vi "rtp play.vi"(4 "voltage range":dbl, 6 "freq":u32, 7 "rtp stop event ref":refnum<user-event>, 8 "error in (no error)":errorcluster caption="에러 입력(에러 없음)", 10 "waveform data":i8[](array[numeric]), 11 "DW7914 입력":refnum<class "DW7914.lvclass">) -> (0 "error out":errorcluster caption="에러 출력", 3 "DW7914 출력":refnum<class "DW7914.lvclass">)   [LabVIEW 2020, in "DW7914.lvclass"]
uses:
  DW7914.lvclass
  Haptic IC/Haptic IC.lvclass/Haptic IC.ctl
  SubVIs/I2C/Instance VIs/(SubVI)I2C_8Bit-8Bit_Read_Single.vi
  SubVIs/I2C/Instance VIs/(SubVI)I2C_8Bit-8Bit_Write_Single.vi
  DW7912/DW7912.lvclass
  Haptic IC/Haptic IC.lvclass
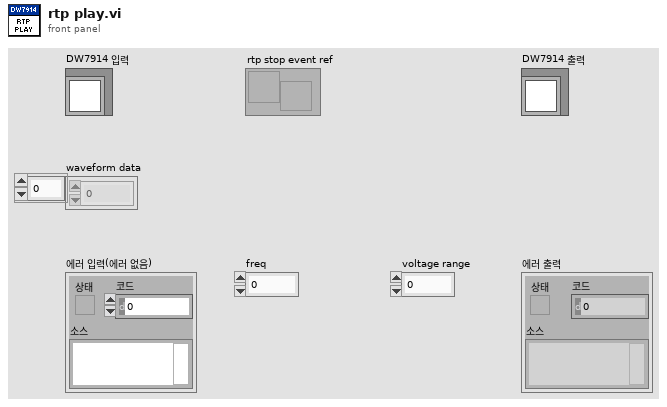
[diagram p1: front panel]
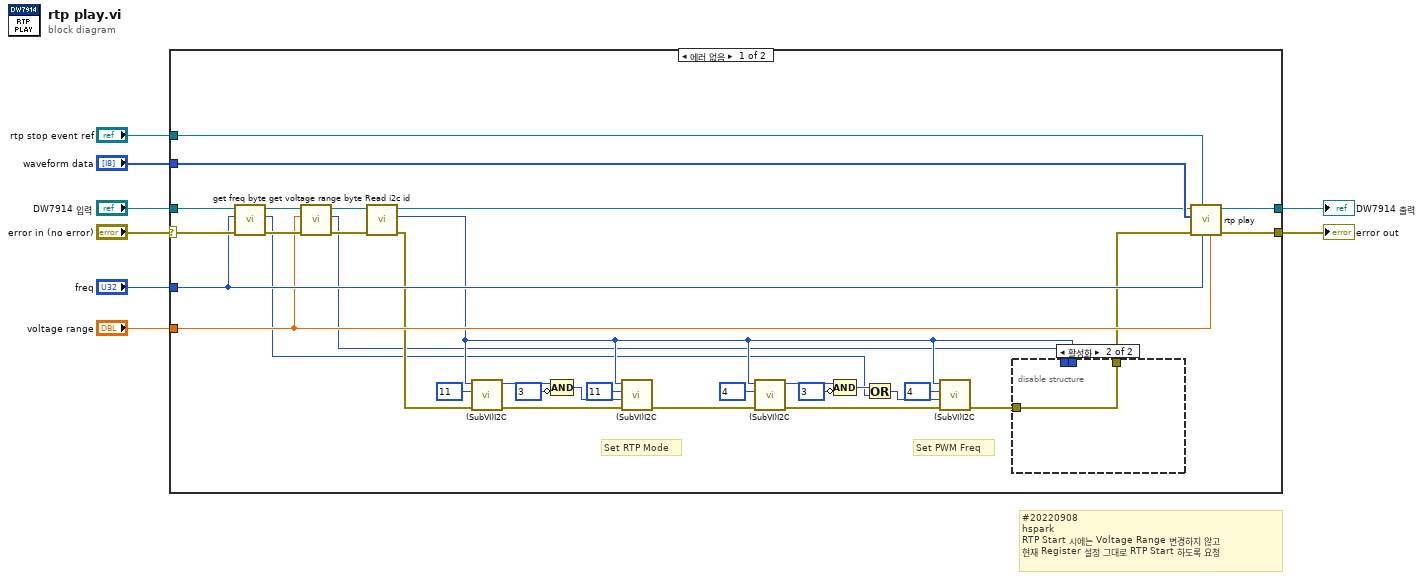
[diagram p0: block diagram]
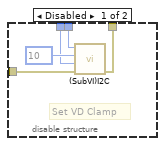
[diagram p2: hidden frame]
diagram:
  # "#20220908\nhspark\nRTP Start 시에는 Voltage Range 변경하지 않고\n현재 Register 설정 그대로 RTP Start 하도록 요청"
  n1 = case shown="에러 없음" "error in (no error)" {
    selector: "error in (no error)" -> [w38 w48]
    tunnel: [w41 w48] -> w8
    tunnel: [w40 w49] -> w7
    tunnel: "voltage range" -> [w32 _]
    tunnel: "freq" -> [w33 _]
    tunnel: "rtp stop event ref" -> [w39 _]
    tunnel: "DW7914 입력" -> [w36 w49]
    tunnel: "waveform data" -> [w37 _]
    frame No Error {
      # "Set PWM Freq"
      # "Set RTP Mode"
      n2 = call-dynamic "get freq byte.vi"("error in (no error)"=w38, "freq"=w33, "DW7912 입력"=w36) -> ("error out"=w35:errorcluster, "byte value"=w10:u8, "DW7912 출력"=w34:refnum<class "DW7914.lvclass">)  [unwired: 6 in]
      n3 = call-dynamic "get voltage range byte.vi"("error in (no error)"=w35, "voltage range"=w32, "DW7912 입력"=w34) -> ("error out"=w31:errorcluster, "byte value"=w9:u8, "DW7912 출력"=w30:refnum<class "DW7914.lvclass">)  [unwired: 6 in]
      n4 = call "Read i2c id.vi"("error in (no error)"=w31, "Haptic IC 입력"=w30) -> ("error out"=w28:errorcluster, "i2c id"=w13:u8, "Haptic IC 출력"=w29:refnum<class "DW7914.lvclass">)  [unwired: 7 in]
      n5 = call-poly "(SubVI)I2C.vi"("error in (no error)"=w28, "Address"=u8 11, "ID"=w13) -> ("error out"=w23:errorcluster, "Read Data"=w26:u8)  [unwired: 6 in, 1 out]
      n6 = Compound Arithmetic op=AND(w26, invert u8 3 ("y")) -> (w22:u8)
      n7 = call-poly "(SubVI)I2C.vi"("error in (no error)"=w23, "Data to Write"=w22, "Address"=u8 11, "ID"=w13) -> ("error out"=w16:errorcluster)  [unwired: 6 in, 1 out]
      n8 = call-poly "(SubVI)I2C.vi"("error in (no error)"=w16, "Address"=u8 4, "ID"=w13) -> ("error out"=w20:errorcluster, "Read Data"=w18:u8)  [unwired: 6 in, 1 out]
      n9 = Compound Arithmetic op=AND(w18, invert u8 3 ("y")) -> (w21:u8)
      n10 = Or(x=w21, y=w10) -> (x .or. y?=w11:u8)
      n11 = call-poly "(SubVI)I2C.vi"("error in (no error)"=w20, "Data to Write"=w11, "Address"=u8 4, "ID"=w13) -> ("error out"=w15:errorcluster)  [unwired: 6 in, 1 out]
      n12 = disable-structure shown="활성화" {
        disable-tunnel: w15 -> [w45 w47]
        disable-tunnel: [w44 w47] -> w14
        disable-tunnel: w13 -> [w43 _]
        disable-tunnel: w9 -> [w42 _]
        frame Disabled {
          # "Set VD Clamp"
          n13 = call-poly "(SubVI)I2C.vi"("error in (no error)"=w45, "Data to Write"=w42, "Address"=u8 10, "ID"=w43) -> ("error out"=w44:errorcluster)  [unwired: 6 in, 1 out]
        }
        frame Enabled {
        }
      }
      n14 = call-parent "rtp play.vi"("voltage range"=w32, "freq"=w33, "rtp stop event ref"=w39, "error in (no error)"=w14, "waveform data"=w37, "DW7912 입력"=w29) -> ("error out"=w41:errorcluster, "DW7912 출력"=w40:refnum<class "DW7914.lvclass">)  [unwired: 4 in]
    }
    frame Error {
    }
  }
  "error out" <- w8
  "DW7914 출력" <- w7
